vi "Close.vi"(8 "error in":errorcluster, 11 "SplashScreen":T1) -> (0 "error out":errorcluster, 3 "SplashScreen out":T1)   [LabVIEW 2013, in "RT Temperature Controller.lvlib" / "splash screen.lvlib"]
uses:
  splash screen.lvlib
  splash screen.ctl
  notifier data.ctl
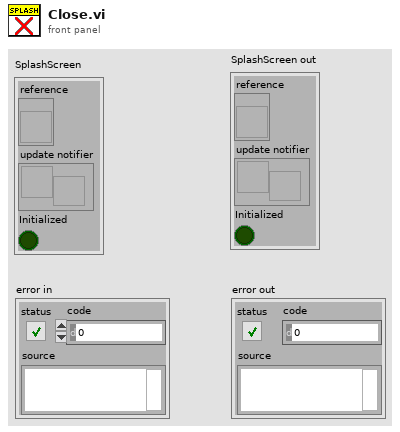
[diagram p1: front panel]
types:
  T1 = typedef "RT Temperature Controller.lvlib/splash screen.lvlib/splash screen.ctl" = cluster{"reference":refnum<vi>, "update notifier":refnum<notifier>, "Initialized":bool}
  T2 = typedef "RT Temperature Controller.lvlib/splash screen.lvlib/notifier data.ctl" = cluster{"Text":string, "percent":dbl}
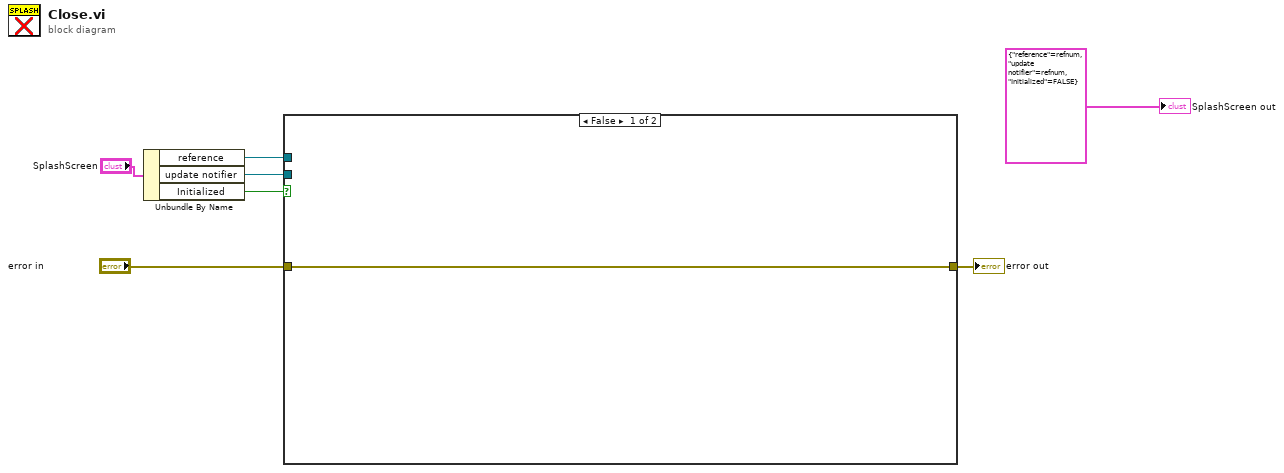
[diagram p0: block diagram]
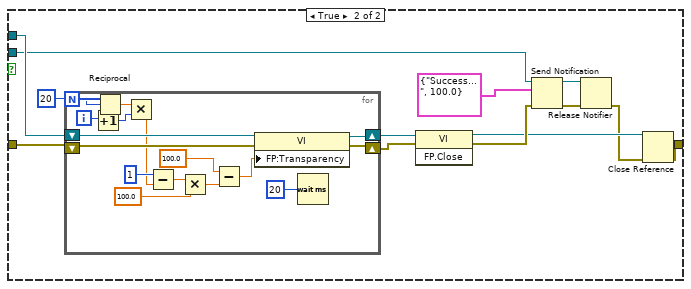
[diagram p2: hidden frame]
diagram:
  n1 = Unbundle By Name("SplashScreen") -> ("reference"=w4:refnum<vi>, "update notifier"=w3:refnum<notifier>, "Initialized"=w1:bool)
  n2 = case shown="False" w1 {
    tunnel: [w8 w18] -> w6
    tunnel: "error in" -> [w8 w16]
    tunnel: w4 -> [_ w15]
    tunnel: w3 -> [_ w14]
    frame False {
    }
    frame True {
      n3 = for {
        N: 20 -> [w31]
        shift-right: [w34] -> w13
        shift-left: w15 -> [w36]
        shift-right: [w37] -> w12
        shift-left: w16 -> [w35]
        i -> [w26]
        n4 = Increment(x=w26) -> (x+1=w25:i32)
        n5 = Reciprocal(x=w31) -> (1/x=w28:dbl)
        n6 = Multiply(x=w28, y=w25) -> (x*y=w27:dbl)
        n7 = Subtract(x=1, y=w27) -> (x-y=w30:dbl)
        n8 = Multiply(x=w30, y=100.0) -> (x*y=w24:dbl)
        n9 = Subtract(x=100.0 ("y"), y=w24) -> (x-y=w22:dbl)
        n10 = property class="VI"(reference=w36, error in=w35, "FP:Transparency"=w22) -> (reference out=w34:refnum<vi>, error out=w37:errorcluster)
        n11 = Wait (ms)(milliseconds to wait=u32 20) -> ()  [unwired: 1 out]
      }
      n12 = invoke class="VI" method="FP.Close"(reference=w13, error in=w12) -> (reference out=w10:refnum<vi>, error out=w11:errorcluster)  [unwired: 1 in, 1 out]
      n13 = Send Notification(notification=T2 {"Text"="Success...", "percent"=100.0}, notifier=w14, error in (no error)=w11) -> (notifier out=w19:refnum<notifier>, error out=w21:errorcluster)
      n14 = Release Notifier(notifier=w19, error in (no error)=w21) -> (error out=w9:errorcluster)  [unwired: 1 in, 2 out]
      n15 = Close Reference(reference=w10, error in (no error)=w9) -> (error out=w18:errorcluster)
    }
  }
  "error out" <- w6
  "SplashScreen out" <- T1 {"reference"=refnum, "update notifier"=refnum, "Initialized"=FALSE} ("SplashScreen out")
